vi "Config Part Information.vi"() -> ()   [LabVIEW 2018]
uses:
  02.Type Def's/All Communication Types.ctl
  type defs/RAP Signal Control.ctl
  type defs/Communication with Motors.ctl
  type defs/EOL Motor Type.ctl
  <vilib>/Utility/config.llb/Write Key (String).vi
  <vilib>/Utility/config.llb/NI_LVConfig.lvlib
panel:
  in  "Turn Off Delay Seconds":u32
  in  "NVH Part Number":u8
  in  "Motor Type":T1
  in  "Send Messages To":T2
  in  "RAP Signal":T3=enum."None"
  in  "Communication Type":T4
  in  "Part Type":string="WK"
  # "Part Configuration"
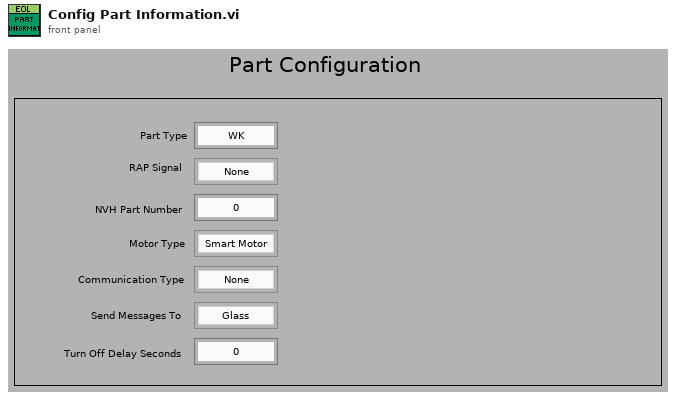
[diagram p1: front panel]
types:
  T1 = typedef "EOL Motor Type.ctl" = enum16{"Smart Motor", "Sensor Motor"}
  T2 = typedef "Communication with Motors.ctl" = enum16{"Glass", "Rollo", "Both"}
  T3 = typedef "RAP Signal Control.ctl" = enum16{"High", "Low", "None"}
  T4 = typedef "All Communication Types.ctl" = enum16{"None", "CAN", "RS 232", "RS 232 LIN", "GM LIN", "SnT LIN", "K Line", "Robel CAN", "P42M-Continental", "Inalfa SCU LIN", "Spare 3"}
  T5 = typedef "NI_LVConfig.lvlib/Config Data RefNum.ctl" = refnum<k1>
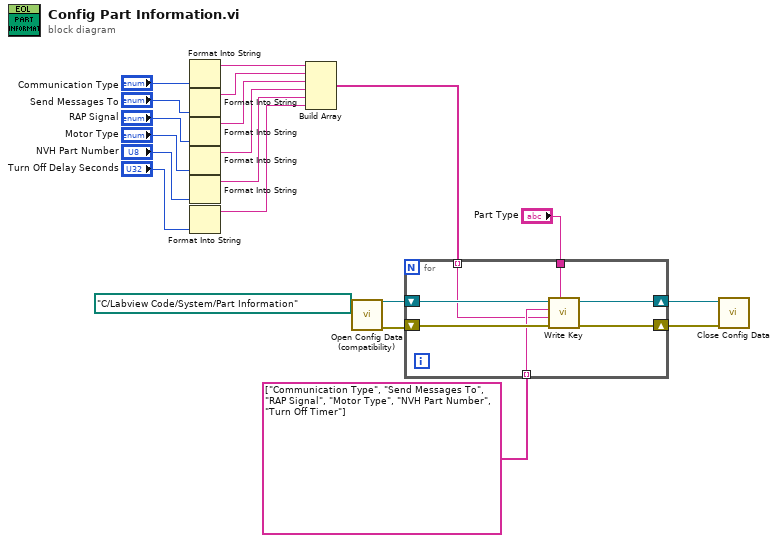
[diagram p0: block diagram]
diagram:
  n1 = Format Into String("Communication Type") -> (resulting string=w8:string)  [unwired: 3 in, 1 out]
  n2 = Format Into String("Send Messages To") -> (resulting string=w7:string)  [unwired: 3 in, 1 out]
  n3 = Format Into String("RAP Signal") -> (resulting string=w6:string)  [unwired: 3 in, 1 out]
  n4 = Format Into String("Motor Type") -> (resulting string=w5:string)  [unwired: 3 in, 1 out]
  n5 = Format Into String("NVH Part Number") -> (resulting string=w4:string)  [unwired: 3 in, 1 out]
  n6 = Format Into String("Turn Off Delay Seconds") -> (resulting string=w1:string)  [unwired: 3 in, 1 out]
  n7 = Build Array(w8, w7, w6, w5, w4, w1) -> (w3:string[])
  n8 = call <vilib>:"Open Config Data (compatibility).vi"("configuration file path"=path "C:/Labview Code/System/Part Information") -> ("error out"=w17:errorcluster, "refnum"=w18:T5)  [unwired: 8 in, 1 out]
  n9 = for {
    tunnel: "Part Type" -> [w27]
    shift-right: [w24] -> w14
    shift-left: w17 -> [w25]
    tunnel: string[] ["Communication Type", "Send Messages To", "RAP Signal", "Motor Type", "NVH Part Number", "Turn Off Timer"] -> [w23] mode=indexing
    shift-right: [w22] -> w15
    shift-left: w18 -> [w26]
    tunnel: w3 -> [w21] mode=indexing
    n10 = call-poly <vilib>:"Write Key.vi"("section"=w27, "error in (no error)"=w25, "value"=w21, "key"=w23, "refnum"=w26) -> ("error out"=w24:errorcluster, "refnum out"=w22:T5)  [unwired: 4 in, 1 out]
  }
  n11 = call <vilib>:"Close Config Data.vi"("error in (no error)"=w14, "refnum"=w15) -> ()  [unwired: 8 in, 2 out]
